vi "DOCK_PRINTER_print_label_manually.vi"(8 "error_in":errorcluster) -> (0 "error_out":errorcluster, 2 "do_printing?":bool, 3 "label_fields_out":T1)   [LabVIEW 2019]
doc: "This VI displays informations about program, contained in about_string, bolding some of the lines in message. If you want to customize look of about message, you can do it here."
uses:
  DOCK_PRINTER_label_fields.ctl
  _misc/AULocalize/SubVIs/RegisterVI.vi
panel:
  out "print_label_header":string caption="Print Label"
  in  "label_fields_in":T1
  in  "cancel":bool
  in  "print":bool
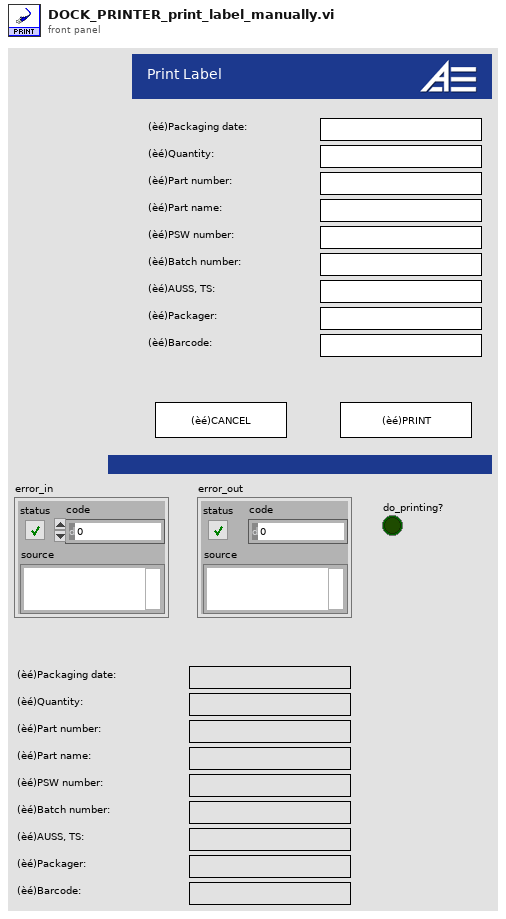
[diagram p1: front panel]
types:
  T1 = typedef "DOCK_PRINTER_label_fields.ctl" = cluster{"packaging_date":string, "quantity":string, "part_number":string, "part_name":string, "PSW_number":string, "batch_number":string, "AUSS, TS":string, "packager":string, "barcode":string}
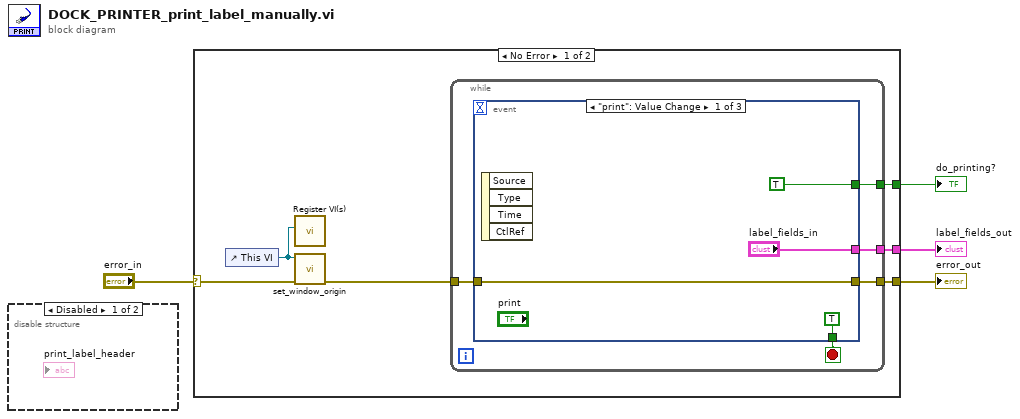
[diagram p0: block diagram]
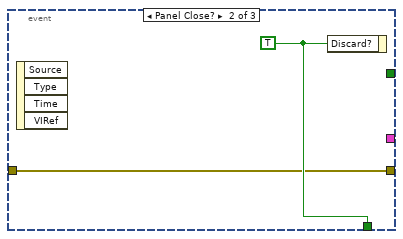
[diagram p3: hidden frame]
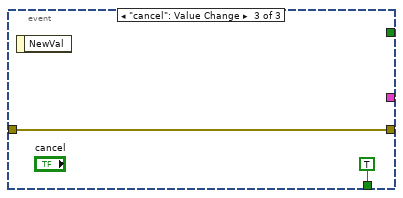
[diagram p4: hidden frame]
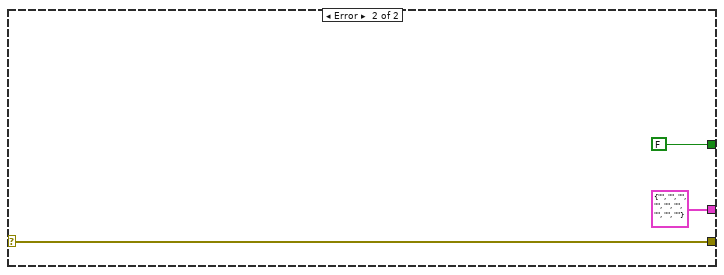
[diagram p5: hidden frame]
diagram:
  n1 = disable-structure shown="Disabled" {
    frame Disabled {
    }
    frame Enabled {
    }
  }
  n2 = case shown="No Error" "error_in" {
    selector: "error_in" -> [w10 w26]
    tunnel: [w8 w26] -> w3
    tunnel: [w7 FALSE ("Discard?")] -> w2
    tunnel: [w6 T1 {"packaging_date"="", "quantity"="", "part_number"="", "part_name"="", "PSW_number"="", "batch_number"="", "AUSS, TS"="", "packager"="", "barcode"=""} ("label_fields_in")] -> w1
    frame No Error {
      n3 = control-ref of="This VI"() -> (w5:refnum<vi>)
      n4 = call-poly "Register VI(s).vi"("VI Ref"=w5) -> ()  [unwired: 9 in, 2 out]
      n5 = call "set_window_origin.vi"("error_in"=w10, "this_vi_reference"=w5) -> ("error_out"=w9:errorcluster)  [unwired: 9 in]
      n6 = while {
        tunnel: w9 -> [w14]
        tunnel: [w13] -> w8
        tunnel: [w12] -> w7
        tunnel: [w11] -> w6
        stop <- w15 stop-if-true
        n7 = event shown="[0] \"print\": Value Change" {
          selector: _ -> [_ _ _]
          dyn-events: _ -> [_ _ _]
          timeout: _ -> [_ _ _]
          tunnel: [TRUE ("stop") w21 TRUE ("Discard?")] -> w15
          tunnel: w14 -> [w18 w20 w23]
          tunnel: [w18 w20 w23] -> w13
          tunnel: [TRUE ("Discard?") _ _] -> w12
          tunnel: ["label_fields_in" _ _] -> w11
          event "print": Value Change {
            n8 = event-data() -> ()  [unwired: 1 in, 4 out]
          }
          event Panel Close? {
            w21 = TRUE ("Discard?")
            n9 = event-data() -> ()  [unwired: 1 in, 4 out]
            n10 = event-data("Discard?"=w21) -> ()  [unwired: 1 in, 1 out]
          }
          event "cancel": Value Change {
            n11 = event-data() -> ()  [unwired: 1 in, 1 out]
          }
        }
      }
    }
    frame Error {
      # "This VI displays informations about program, contained in about_string, bolding some of the lines in message. If you want to customize look of about message, you can do it here."
    }
  }
  "error_out" <- w3
  "do_printing?" <- w2
  "label_fields_out" <- w1
